vi "Modules Edit.vi"(6 "Queue Ref":T1={"UI"=refnum, "Message"=refnum, "Data"=refnum, "Caller"=refnum, "Name"="000 Common", "Data Path"=path "", "Class Path"=path "", "SubPanel"=refnum, "Project Name"="", "MNT"="", "Title"="", "Data Source"=refnum, "Queue List"={}, "VI"=refnum, "UE"=refnum}, 8 "error in (no error)":errorcluster caption="Error In", 9 "Data":variant, 10 "Operate":string, 11 "ModulesRef":refnum<vi>) -> (0 "error out":errorcluster caption="Error Out")   [LabVIEW 2020]
uses:
  Alin/QMH/000 Module Data Type.ctl
  Alin/QMH/Queue Message.ctl
  0007 Controls/Data Module.ctl
  0007 Controls/Data Modules.ctl
  0007 Controls/Data Element Single.ctl
  Global/Data Global/SDQ Data Type.ctl
  6af73d8b-4b54-4092-88b9-52990f3e3bae.vi
  94913dd2-90ff-4ca1-8781-ffadfa0ced3e.vi
  d649981d-6ad0-461c-86a9-d94ae38d726b.vi
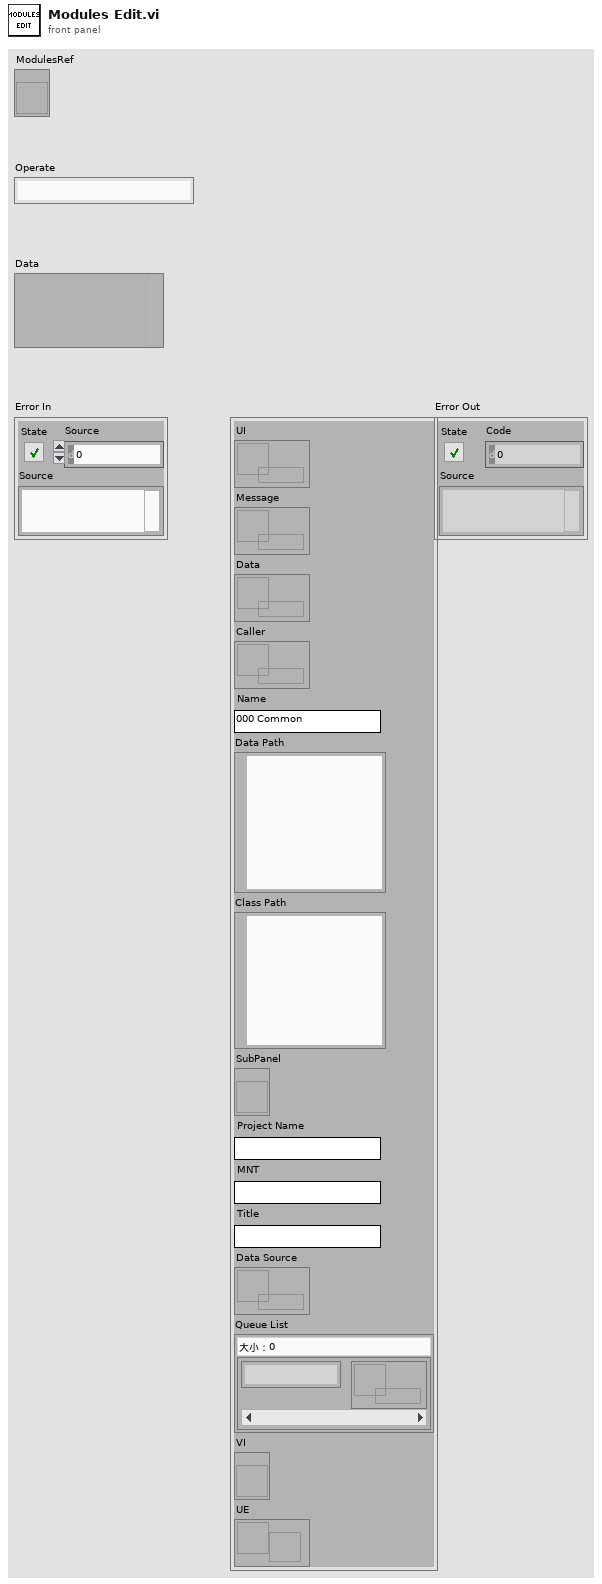
[diagram p1: front panel]
types:
  T1 = typedef "000 Module Data Type.ctl" = cluster{"UI":refnum<queue>, "Message":refnum<queue>, "Data":refnum<queue>, "Caller":refnum<queue>, "Name":string, "Data Path":path, "Class Path":path, "SubPanel":refnum<vi>, "Project Name":string, "MNT":string, "Title":string, "Data Source":refnum<queue>, "Queue List":map{string, refnum<queue>}, "VI":refnum<vi>, "UE":refnum<user-event>}
  T2 = typedef "SDQ Data Type.ctl" = cluster{"CAN Length":string, "CAN Name":string, "CAN ID":string, "CAN Type":string, "Test Item":string, "Byte Order":string, "Instruction":string, "Control Type":string, "Group":string, "Offset":dbl, "Coefficient":dbl, "Write Enable":bool, "Lable Type":string, "Key?":string, "Set Value":string, "Upper":dbl, "Lower":dbl, "Unit":string, "Formula":string, "Test Item Type":string, "Length":i32, "Address":string, "Name":string, "Identifier":string, "Data Type":string, "Enumerate?":string, "Enumerate List":string, "Data":string, "Source":string}
  T3 = cluster{"Receive Data":map{string, T2}, "Queue Ref":T1, "Digit":dbl, "ModulesRef":refnum<vi>, "Index":cluster{"Row":i32, "Colcum":i32, "Digit":dbl}, "Last Index":cluster{"Row":i32, "Colcum":i32, "Digit":dbl}}
  T4 = typedef "Data Module.ctl" = cluster{"Module01":T5, "Module02":T5, "Module03":T5, "Module04":T5, "Module05":T5, "Module06":T5, "Module07":T5, "Module08":T5, "Module09":T5, "Module10":T5, "Module11":T5}
  T5 = typedef "Data Modules.ctl" = cluster{"Names":cluster{"Module Name":string, "Set Value":string, "Real Value":string, "FB Value":string, "Unit":string, "Identifier":string, "IdentifierW":string, "Decimal":string, "AS":bool, "AR":bool, "Con":bool}, "Data":T6[], "Digit":dbl}
  T6 = typedef "Data Element Single.ctl" = cluster{"Name":string, "Set Value":string, "Real Value":string, "FB Value":string, "Unit":string, "Identifier":string, "Write Name":string, "Decimal":u16, "AS":bool, "AR":bool, "ALM":bool, "Up":bool, "Down":bool}
  T7 = cluster{"输出簇":cluster{i32, i32, "Digit":dbl}, "Modules":T4}
  T8 = cluster{"Modules[0]":T5, "Modules[1]":T5, "Modules[2]":T5, "Modules[3]":T5, "Modules[4]":T5, "Modules[5]":T5, "Modules[6]":T5, "Modules[7]":T5, "Modules[8]":T5, "Modules[9]":T5, "Modules[10]":T5}
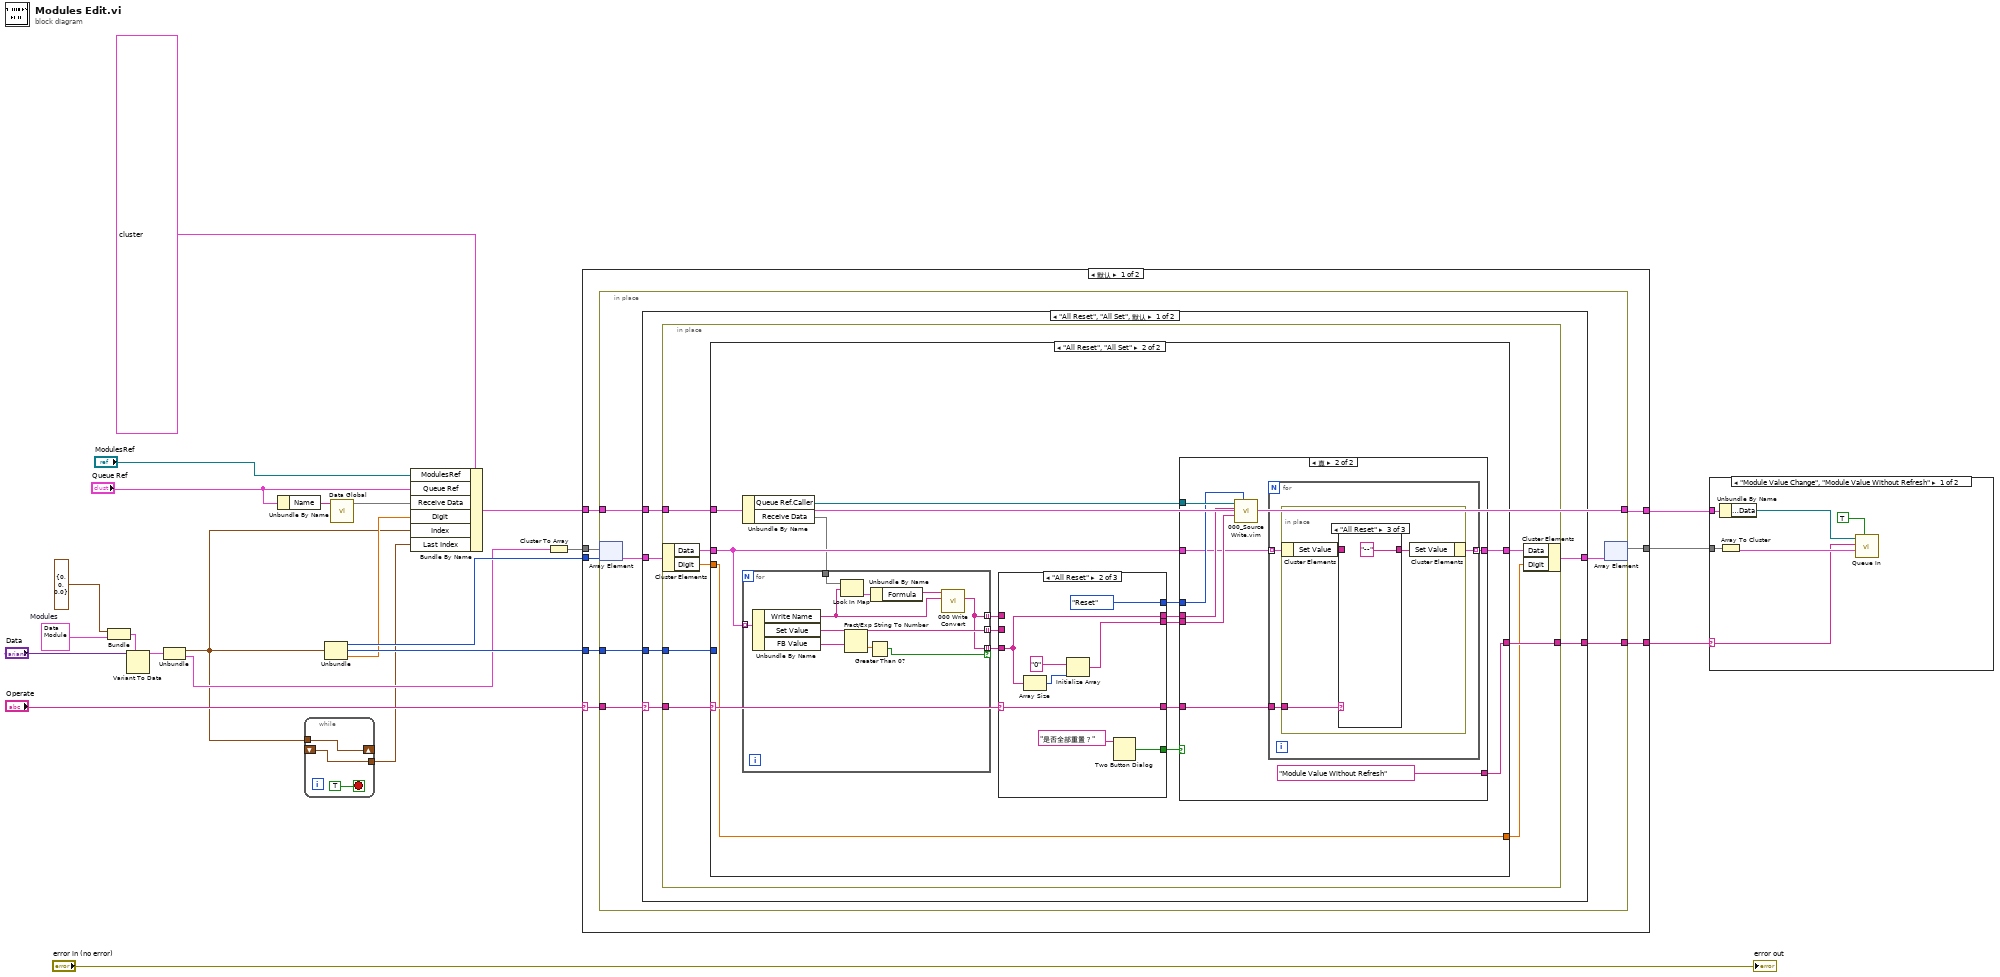
[diagram p0: block diagram]
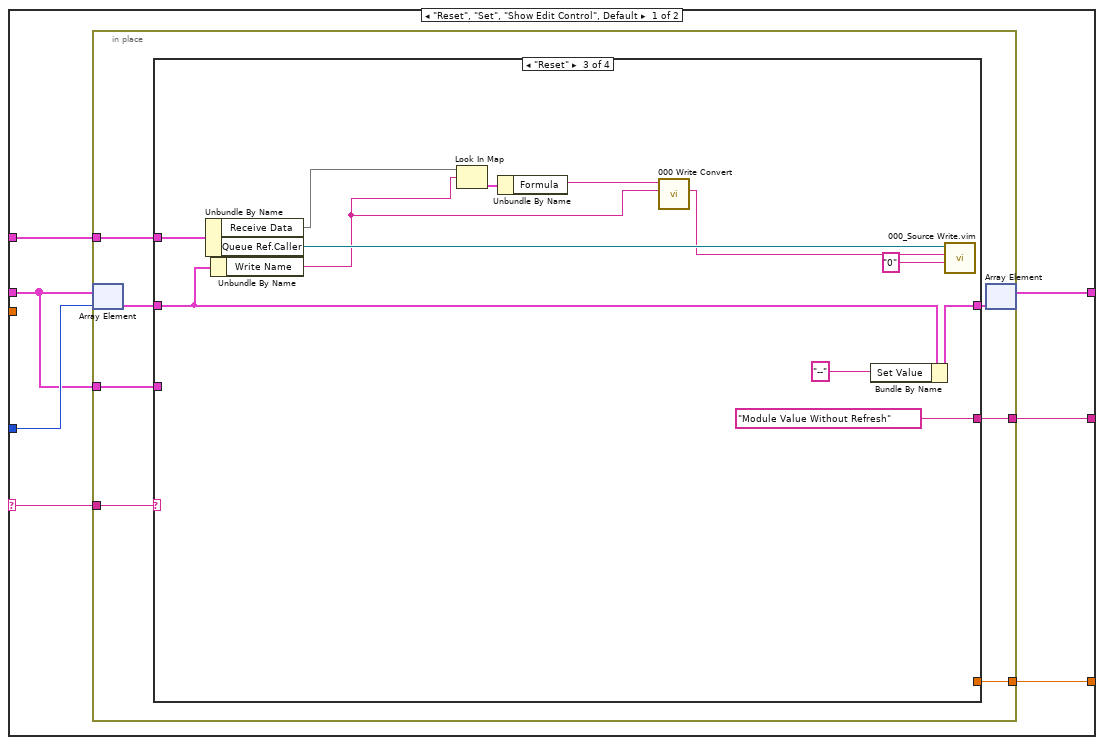
[diagram p2: hidden frame]
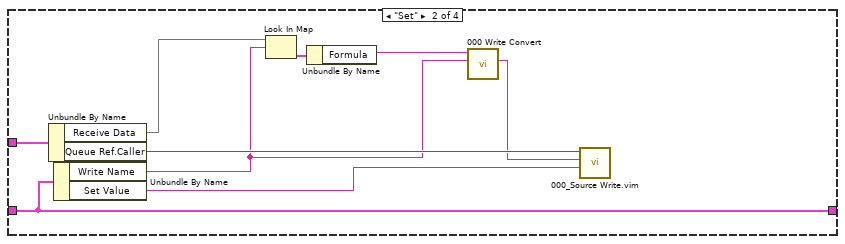
[diagram p4: hidden frame]
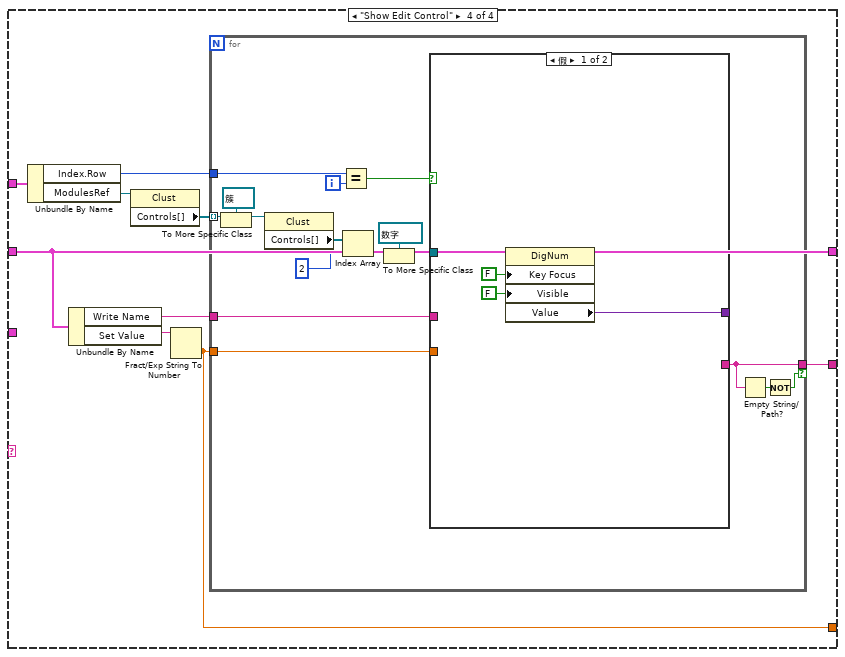
[diagram p5: hidden frame]
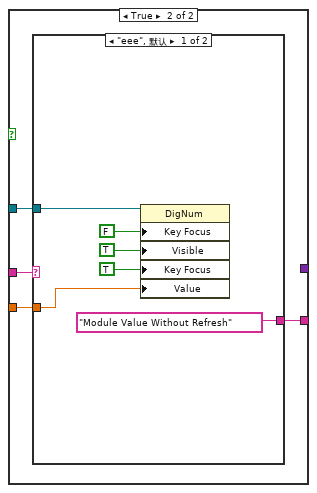
[diagram p6: hidden frame]
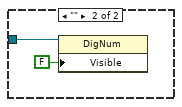
[diagram p7: hidden frame]
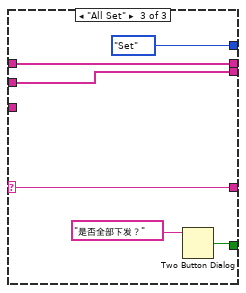
[diagram p12: hidden frame]
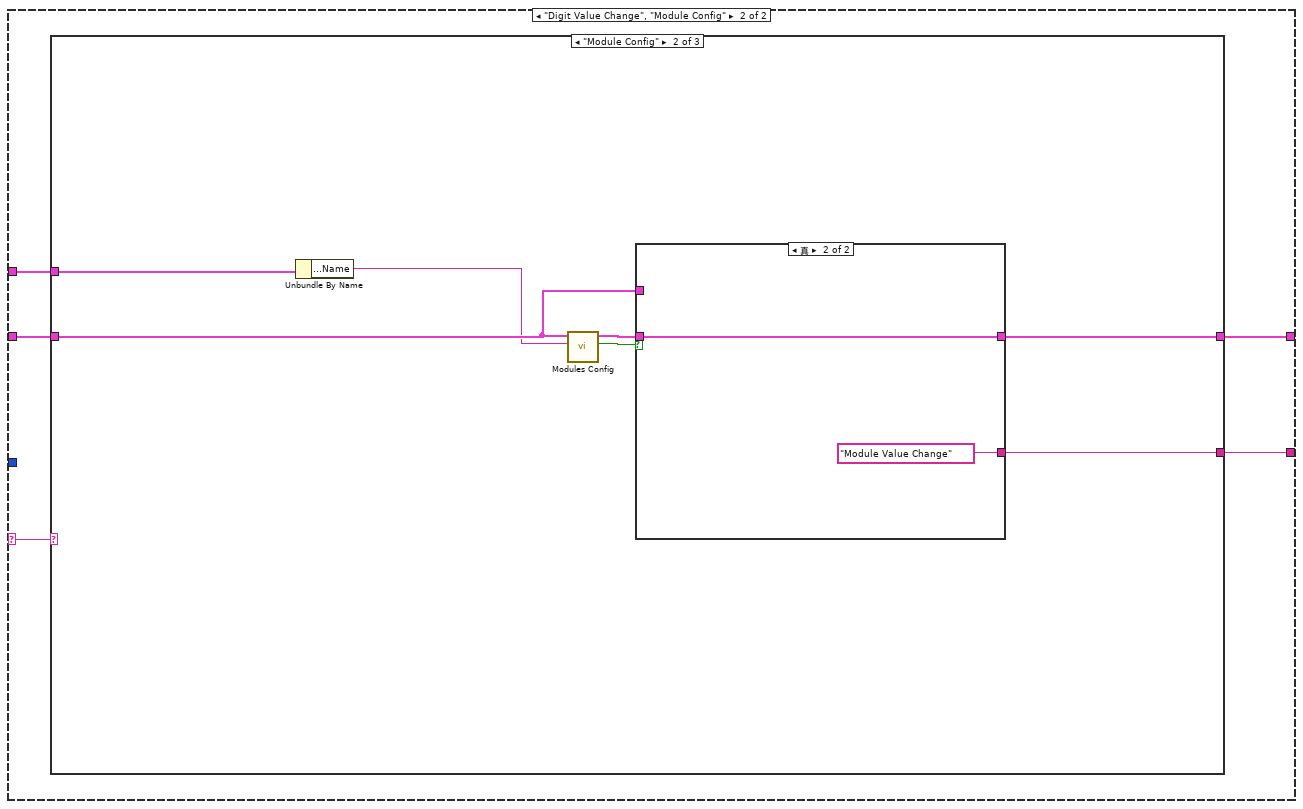
[diagram p13: hidden frame]
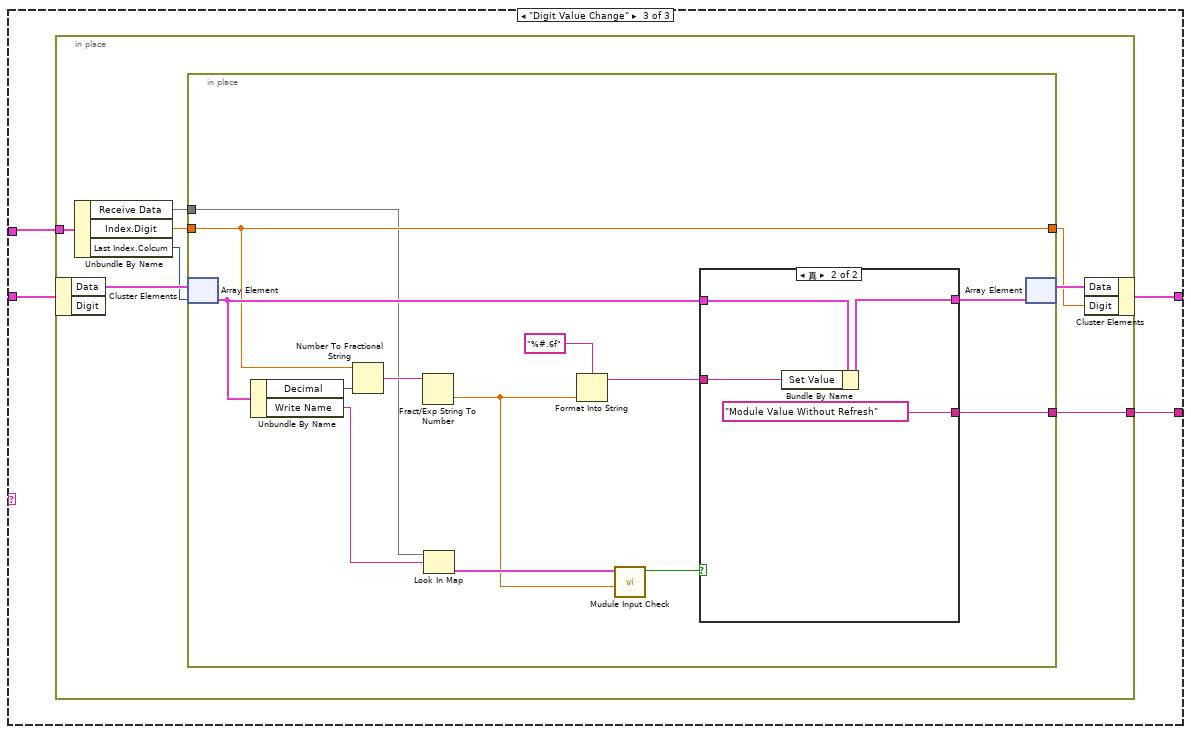
[diagram p16: hidden frame]
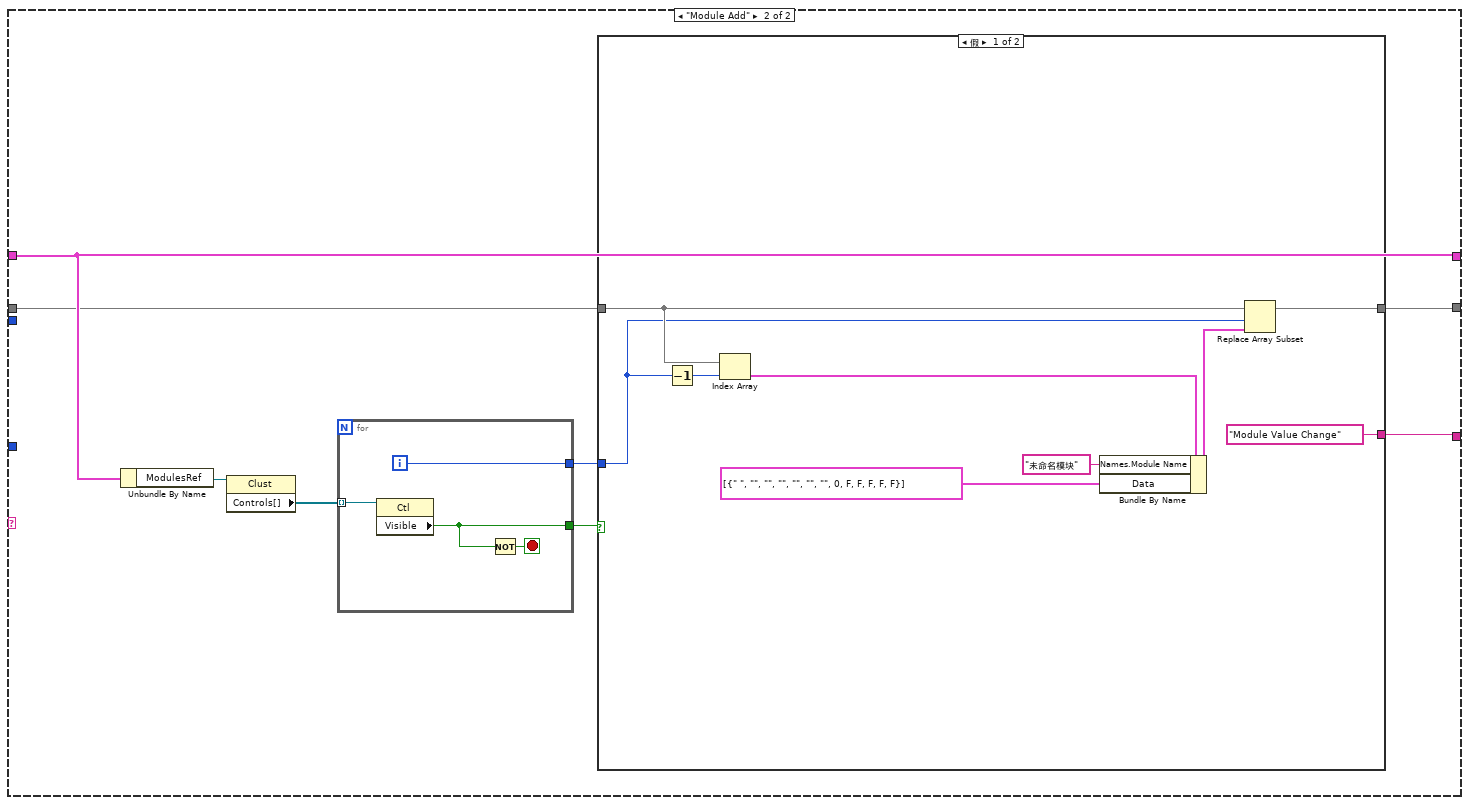
[diagram p18: hidden frame]
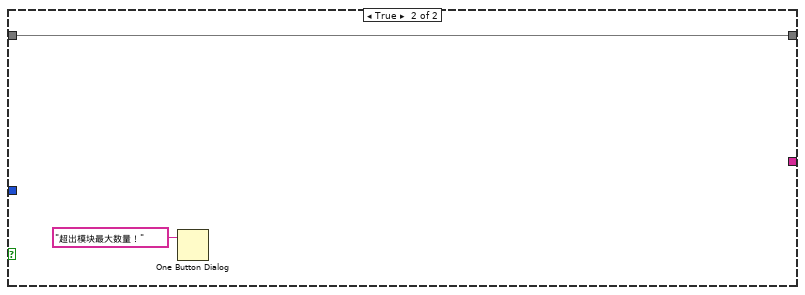
[diagram p19: hidden frame]
diagram:
  w13 = T4 {"Module01"={"Names"={"Module Name"="", "Set Value"="", "Real Value"="", "FB Value"="", "Unit"="", "Identifier"="", "IdentifierW"="写入标识符", "Decimal"="位数", "AS"=FALSE, "AR"=FALSE, "Con"=FALSE}, "Data"=[], "Digit"=0.0}, "Module02"={"Names"={"Module Name"="", "Set Value"="", "Real Value"="", "FB Value"="", "Unit"="", "Identifier"="", "IdentifierW"="写入标识符", "Decimal"="位数", "AS"=FALSE, "AR"=FALSE, "Con"=FALSE}, "Data"=[], "Digit"=0.0}, "Module03"={"Names"={"Module Name"="", "Set Value"="", "Real Value"="", "FB Value"="", "Unit"="", "Identifier"="", "IdentifierW"="写入标识符", "Decimal"="位数", "AS"=FALSE, "AR"=FALSE, "Con"=FALSE}, "Data"=[], "Digit"=0.0}, "Module04"={"Names"={"Module Name"="", "Set Value"="", "Real Value"="", "FB Value"="", "Unit"="", "Identifier"="", "IdentifierW"="写入标识符", "Decimal"="位数", "AS"=FALSE, "AR"=FALSE, "Con"=FALSE}, "Data"=[], "Digit"=0.0}, "Module05"={"Names"={"Module Name"="", "Set Value"="", "Real Value"="", "FB Value"="", "Unit"="", "Identifier"="", "IdentifierW"="写入标识符", "Decimal"="位数", "AS"=FALSE, "AR"=FALSE, "Con"=FALSE}, "Data"=[], "Digit"=0.0}, "Module06"={"Names"={"Module Name"="", "Set Value"="", "Real Value"="", "FB Value"="", "Unit"="", "Identifier"="", "IdentifierW"="写入标识符", "Decimal"="位数", "AS"=FALSE, "AR"=FALSE, "Con"=FALSE}, "Data"=[], "Digit"=0.0}, "Module07"={"Names"={"Module Name"="", "Set Value"="", "Real Value"="", "FB Value"="", "Unit"="", "Identifier"="", "IdentifierW"="写入标识符", "Decimal"="位数", "AS"=FALSE, "AR"=FALSE, "Con"=FALSE}, "Data"=[], "Digit"=0.0}, "Module08"={"Names"={"Module Name"="", "Set Value"="", "Real Value"="", "FB Value"="", "Unit"="", "Identifier"="", "IdentifierW"="写入标识符", "Decimal"="位数", "AS"=FALSE, "AR"=FALSE, "Con"=FALSE}, "Data"=[], "Digit"=0.0}, "Module09"={"Names"={"Module Name"="", "Set Value"="", "Real Value"="", "FB Value"="", "Unit"="", "Identifier"="", "IdentifierW"="写入标识符", "Decimal"="位数", "AS"=FALSE, "AR"=FALSE, "Con"=FALSE}, "Data"=[], "Digit"=0.0}, "Module10"={"Names"={"Module Name"="", "Set Value"="", "Real Value"="", "FB Value"="", "Unit"="", "Identifier"="", "IdentifierW"="写入标识符", "Decimal"="位数", "AS"=FALSE, "AR"=FALSE, "Con"=FALSE}, "Data"=[], "Digit"=0.0}, "Module11"={"Names"={"Module Name"="", "Set Value"="", "Real Value"="", "FB Value"="", "Unit"="", "Identifier"="", "IdentifierW"="写入标识符", "Decimal"="位数", "AS"=FALSE, "AR"=FALSE, "Con"=FALSE}, "Data"=[], "Digit"=0.0}}  # Modules
  n1 = Bundle("输出簇"=cluster{i32, i32, "Digit":dbl} {0, 0, "Digit"=0.0}, "Modules"=w13) -> (w12:T7)  [unwired: 1 in]
  n2 = Variant To Data(type=w12, Variant="Data") -> (data=w14:T7)  [unwired: 1 in, 1 out]
  n3 = Unbundle(w14) -> ("输出簇"=w2:cluster{i32, i32, "Digit":dbl}, "Modules"=w7:T4)
  n4 = Unbundle By Name("Queue Ref") -> ("Name"=w5:string)
  n5 = while {
    shift-right: [w26] -> _
    shift-left: _ -> [w24]
    tunnel: w2 -> [w26]
    tunnel: [w24] -> w1
    stop <- TRUE stop-if-true
  }
  n6 = Unbundle(w2) -> (w16:i32, w19:i32, "Digit"=w3:dbl)
  n7 = call "Data Global.vi"("Name"=w5) -> ("Data Out"=w4:map{string, T2})  [unwired: 7 in, 3 out]
  n8 = Bundle By Name(cluster=T3 {"Receive Data"={}, "Queue Ref"={"UI"=refnum, "Message"=refnum, "Data"=refnum, "Caller"=refnum, "Name"="0001_HZKD_ST01-DSM-002_DataMonitor", "Data Path"=path "D:/NBT/01-Project/02-Processing/NBT-TestPlatform V2/NBT-TestPlatform 20230413_0/Config/NBT/NBT_V1.0.0/Project/0001_HZKD_ST01/04_DataUse/002_DataMonitor.csv", "Class Path"=path "D:/NBT/01-Project/02-Processing/NBT-TestPlatform V2/NBT-TestPlatform 20230413_0/Modules/000 UI/002_Module/002_DataMonitor.vi", "SubPanel"=refnum, "Project Name"="0001_HZKD_ST01", "MNT"="", "Title"="", "Data Source"=refnum, "Queue List"={}, "VI"=refnum, "UE"=refnum}, "Digit"=0.0, "ModulesRef"=refnum, "Index"={"Row"=0, "Colcum"=0, "Digit"=0.0}, "Last Index"={"Row"=0, "Colcum"=0, "Digit"=0.0}}, "ModulesRef"="ModulesRef", "Queue Ref"="Queue Ref", "Receive Data"=w4, "Digit"=w3, "Index"=w2, "Last Index"=w1) -> (w10:T3)
  n9 = Cluster To Array(cluster=w7) -> (array=w23:T5[])
  n10 = case shown="默认" "Operate" {
    selector: "Operate" -> [w31 _]
    tunnel: w23 -> [w34 w239]
    tunnel: [w33 w238] -> w21
    tunnel: w19 -> [w32 _]
    tunnel: w16 -> [w30 _]
    tunnel: w10 -> [w29 w244]
    tunnel: [w28 w244] -> w9
    tunnel: [w27 w237] -> w8
    frame Default {
      n11 = in-place {
        in-place-border: w32 -> [w40]
        in-place-border: w31 -> [w38]
        in-place-border: w29 -> [w37]
        in-place-border: [w37] -> w28
        in-place-border: [w35] -> w27
        n12 = in-place-array #1(w34, w30) -> (w36:T5)
        n13 = case shown="\"All Reset\", \"All Set\", 默认" w38 {
          selector: w38 -> [w44 w192]
          tunnel: w40 -> [w46 _]
          tunnel: [w45 w194] -> w39
          tunnel: w37 -> [w43 w195]
          tunnel: w36 -> [w42 w193]
          tunnel: [w41 w191] -> w35
          frame "All Reset", "All Set", Default {
            n14 = in-place {
              in-place-border: w46 -> [w54]
              in-place-border: w44 -> [w52]
              in-place-border: w43 -> [w49]
              in-place-border: [w48] -> w41
              n15 = in-place-cluster #2(w42) -> ("Data"=w51:T6[], "Digit"=w50:dbl)
              n16 = case shown="\"All Reset\", \"All Set\"" w52 {
                selector: w52 -> [w59 w145]
                tunnel: w54 -> [w61 _]
                tunnel: [w60 w138] -> w53
                tunnel: w51 -> [w58 w139]
                tunnel: w50 -> [_ w135]
                tunnel: w49 -> [w57 w147]
                tunnel: [w56 w136] -> w48
                tunnel: [w55 w135] -> w47
                frame "Reset", "Set", "Show Edit Control", Default {
                  n17 = in-place {
                    in-place-border: w59 -> [w67]
                    in-place-border: w58 -> [w65]
                    in-place-border: w57 -> [w64]
                    in-place-border: [w63] -> w56
                    in-place-border: [w62] -> w55
                    n18 = in-place-array #3(w58, w61) -> (w68:T6)
                    n19 = case shown="\"Reset\"" w67 {
                      tunnel: w68 -> [w69 w76 w85 w95]
                      tunnel: [w69 w76 w90 w95] -> w66
                      tunnel: w65 -> [_ _ _ _]
                      tunnel: w64 -> [_ w78 w86 w99]
                      tunnel: [_ _ "Module Value Without Refresh" w91] -> w63
                      tunnel: [_ _ _ w92] -> w62
                      frame "eee", Default {
                      }
                      frame "Set" {
                        n20 = Unbundle By Name(w78) -> ("Receive Data"=w74:map{string, T2}, "Queue Ref.Caller"=w77:refnum<queue>)
                        n21 = Unbundle By Name(w76) -> ("Write Name"=w71:string, "Set Value"=w75:string)
                        n22 = Look In Map(map=w74, key=w71) -> (value=w73:T2)  [unwired: 1 in, 1 out]
                        n23 = Unbundle By Name(w73) -> ("Formula"=w72:string)
                        n24 = call "000 Write Convert.vi"("Name In"=w71, "Formular"=w72) -> ("Name Out"=w70:string)  [unwired: 9 in]
                        n25 = call "000_Source Write.vim"("Data"=w75, "Name"=w70, "Queue In"=w77) -> ()  [unwired: 6 in, 3 out]
                      }
                      frame "Reset" {
                        n26 = Unbundle By Name(w86) -> ("Receive Data"=w81:map{string, T2}, "Queue Ref.Caller"=w87:refnum<queue>)
                        n27 = Unbundle By Name(w85) -> ("Write Name"=w80:string)
                        n28 = Look In Map(map=w81, key=w80) -> (value=w83:T2)  [unwired: 1 in, 1 out]
                        n29 = Unbundle By Name(w83) -> ("Formula"=w82:string)
                        n30 = call "000 Write Convert.vi"("Name In"=w80, "Formular"=w82) -> ("Name Out"=w79:string)  [unwired: 9 in]
                        n31 = Bundle By Name(cluster=w85, "Set Value"="--") -> (w90:T6)
                        n32 = call "000_Source Write.vim"("Data"="0", "Name"=w79, "Queue In"=w87) -> ()  [unwired: 6 in, 3 out]
                      }
                      frame "Show Edit Control" {
                        n33 = Unbundle By Name(w99) -> ("Index.Row"=w96:i32, "ModulesRef"=w98:refnum<vi>)
                        n34 = Unbundle By Name(w95) -> ("Write Name"=w93:string, "Set Value"=w94:string)
                        n35 = property class="Clust"(reference=w98) -> ("Controls[]"=w97:refnum<vi>[])  [unwired: 1 in, 2 out]
                        n36 = Fract/Exp String To Number(string=w94) -> (number=w92:dbl)  [unwired: 3 in, 1 out]
                        n37 = for {
                          tunnel: w97 -> [w111] mode=indexing
                          tunnel: w96 -> [w109]
                          tunnel: w92 -> [w105]
                          tunnel: w93 -> [w103]
                          tunnel: [w102] -> w91 if=w100
                          i -> [w108]
                          n38 = To More Specific Class(target class=refnum<vi> refnum ("ModulesRef"), reference=w111) -> (specific class reference=w115:refnum<vi>)  [unwired: 1 in, 1 out]
                          n39 = property class="Clust"(reference=w115) -> ("Controls[]"=w114:refnum<vi>[])  [unwired: 1 in, 2 out]
                          n40 = Equal?(x=w109, y=w108) -> (x = y?=w107:bool)
                          n41 = Index Array(array=w114, index=2 ("索引")) -> (element=w110:refnum<vi>)
                          n42 = To More Specific Class(target class=refnum<vi> refnum ("Digit"), reference=w110) -> (specific class reference=w106:refnum<vi>)  [unwired: 1 in, 1 out]
                          n43 = case shown="假" w107 {
                            tunnel: w106 -> [w119 w123]
                            tunnel: w105 -> [_ w122]
                            tunnel: w103 -> [_ w121]
                            tunnel: [_ w120] -> w102
                            tunnel: [w116 _] -> _
                            frame False {
                              n44 = property class="DigNum"(reference=w119, "Key Focus"=FALSE ("键选中"), "Visible"=FALSE ("可见")) -> ("Value"=w116:variant)  [unwired: 1 in, 2 out]
                            }
                            frame True {
                              n45 = case shown="\"eee\", 默认" w121 {
                                tunnel: w123 -> [w127 w130]
                                tunnel: w122 -> [w126 _]
                                tunnel: ["Module Value Without Refresh" _] -> w120
                                frame "eee", Default {
                                n46 = property class="DigNum"(reference=w127, "Key Focus"=FALSE ("键选中"), "Visible"=TRUE ("可见"), "Key Focus"=TRUE ("键选中"), "Value"=w126) -> ()  [unwired: 1 in, 2 out]
                                }
                                frame "" {
                                n47 = property class="DigNum"(reference=w130, "Visible"=FALSE ("可见")) -> ()  [unwired: 1 in, 2 out]
                                }
                              }
                            }
                          }
                          n48 = Empty String/Path?(string/path=w102) -> (empty?=w101:bool)
                          n49 = Not(x=w101) -> (.not. x?=w100:bool)
                        }
                      }
                    }
                    n50 = in-place-array #3(w66) -> (w60:T6[])  [unwired: 1 out]
                  }
                }
                frame "All Reset", "All Set" {
                  n51 = Unbundle By Name(w147) -> ("Queue Ref.Caller"=w146:refnum<queue>, "Receive Data"=w133:map{string, T2})
                  n52 = for {
                    tunnel: w139 -> [w190] mode=indexing
                    tunnel: [w181] -> w144 mode=indexing
                    tunnel: [w183] -> w143 mode=indexing
                    tunnel: [w181] -> w134 mode=indexing if=w188
                    tunnel: w133 -> [w184]
                    n53 = Unbundle By Name(w190) -> ("Write Name"=w182:string, "Set Value"=w183:string, "FB Value"=w187:string)
                    n54 = Look In Map(map=w184, key=w182) -> (value=w186:T2)  [unwired: 1 in, 1 out]
                    n55 = Fract/Exp String To Number(string=w187) -> (number=w189:dbl)  [unwired: 3 in, 1 out]
                    n56 = Greater Than 0?(x=w189) -> (x > 0?=w188:bool)
                    n57 = Unbundle By Name(w186) -> ("Formula"=w185:string)
                    n58 = call "000 Write Convert.vi"("Name In"=w182, "Formular"=w185) -> ("Name Out"=w181:string)  [unwired: 9 in]
                  }
                  n59 = case shown="\"All Reset\"" w145 {
                    selector: w145 -> [w166 w170 w177]
                    tunnel: w144 -> [_ _ w180]
                    tunnel: w143 -> [_ _ w179]
                    tunnel: [_ w169 w180] -> w142
                    tunnel: [_ w172 w179] -> w141
                    tunnel: [_ enum16{"Set", "Reset"}."Reset" ("Operate") enum16{"Set", "Reset"}."Set" ("Operate")] -> w140
                    tunnel: [w166 w170 w177] -> w137
                    tunnel: w134 -> [_ w169 _]
                    tunnel: [_ w167 w176] -> w132
                    frame "eee", Default {
                    }
                    frame "All Reset" {
                      n60 = Array Size(array=w169) -> (size(s)=w173:i32)
                      n61 = Initialize Array("0", w173) -> (w172:string[])
                      n62 = Two Button Dialog(message="是否全部重置？") -> (T button?=w167:bool)  [unwired: 2 in]
                    }
                    frame "All Set" {
                      n63 = Two Button Dialog(message="是否全部下发？") -> (T button?=w176:bool)  [unwired: 2 in]
                    }
                  }
                  n64 = case shown="真" w132 {
                    tunnel: w146 -> [_ w156]
                    tunnel: w142 -> [_ w155]
                    tunnel: w141 -> [_ w154]
                    tunnel: w140 -> [_ w153]
                    tunnel: w139 -> [w148 w152]
                    tunnel: [w148 w151] -> w138
                    tunnel: w137 -> [_ w150]
                    tunnel: [_ "Module Value Without Refresh"] -> w136
                    frame False {
                    }
                    frame True {
                      n65 = call "000_Source Write.vim"("Operate"=w153, "Data"=w154, "Name"=w155, "Queue In"=w156) -> ()  [unwired: 5 in, 3 out]
                      n66 = for {
                        tunnel: w152 -> [w159] mode=indexing
                        tunnel: [w158] -> w151 mode=indexing
                        tunnel: w150 -> [w157]
                        n67 = in-place {
                          in-place-border: w157 -> [w162]
                          n68 = in-place-cluster #4(w159) -> ("Set Value"=w161:string)
                          n69 = case shown="\"All Reset\"" w162 {
                            tunnel: w161 -> [w163 w164 _]
                            tunnel: [w163 w164 "--" ("Name")] -> w160
                            frame "eee", Default {
                            }
                            frame "All Set" {
                            }
                            frame "All Reset" {
                            }
                          }
                          n70 = in-place-cluster #4("Set Value"=w160) -> (w158:T6)
                        }
                      }
                    }
                  }
                }
              }
              n71 = in-place-cluster #2("Data"=w53, "Digit"=w47) -> (w45:T5)
            }
          }
          frame "Digit Value Change", "Module Config" {
            n72 = case shown="\"Module Config\"" w192 {
              tunnel: w195 -> [_ w203 w208]
              tunnel: [w196 w200 w209] -> w194
              tunnel: w193 -> [w196 w199 w210]
              tunnel: [_ w198 w207] -> w191
              frame "eee", Default {
              }
              frame "Module Config" {
                n73 = Unbundle By Name(w203) -> ("Queue Ref.Name"=w197:string)
                n74 = call "Modules Config.vi"("Name"=w197, "Module In"=w199) -> ("OK？"=w202:bool, "Module Out"=w201:T5)  [unwired: 8 in]
                n75 = case shown="真" w202 {
                  tunnel: w201 -> [_ w206]
                  tunnel: [w204 w206] -> w200
                  tunnel: w199 -> [w204 _]
                  tunnel: [_ "Module Value Change"] -> w198
                  frame False {
                  }
                  frame True {
                  }
                }
              }
              frame "Digit Value Change" {
                n76 = in-place {
                  in-place-border: w208 -> [w217]
                  in-place-border: [w213] -> w207
                  n77 = in-place-cluster #5(w210) -> ("Data"=w218:T6[])  [unwired: 1 out]
                  n78 = Unbundle By Name(w217) -> ("Receive Data"=w211:map{string, T2}, "Index.Digit"=w215:dbl, "Last Index.Colcum"=w216:i32)
                  n79 = in-place {
                    in-place-border: w215 -> [w227]
                    in-place-border: [w229] -> w213
                    in-place-border: [w227] -> w212
                    in-place-border: w211 -> [w223]
                    n80 = in-place-array #6(w218, w216) -> (w231:T6)
                    n81 = Unbundle By Name(w231) -> ("Decimal"=w226:u16, "Write Name"=w222:string)
                    n82 = Number To Fractional String(number=w227, precision (6)=w226) -> (F-format string=w225:string)  [unwired: 2 in]
                    n83 = Fract/Exp String To Number(string=w225) -> (number=w220:dbl)  [unwired: 3 in, 1 out]
                    n84 = Look In Map(map=w223, key=w222) -> (value=w221:T2)  [unwired: 1 in, 1 out]
                    n85 = Format Into String(format string="%#.6f" ("格式字符串"), w220) -> (resulting string=w224:string)  [unwired: 2 in, 1 out]
                    n86 = call "Mudule Input Check.vi"("Data In"=w220, "Value"=w221) -> ("OK?"=w219:bool)  [unwired: 9 in]
                    n87 = case shown="真" w219 {
                      tunnel: w231 -> [w232 w236]
                      tunnel: [w232 w235] -> w230
                      tunnel: [_ "Module Value Without Refresh"] -> w229
                      tunnel: w224 -> [_ w233]
                      frame False {
                      }
                      frame True {
                        n88 = Bundle By Name(cluster=w236, "Set Value"=w233) -> (w235:T6)
                      }
                    }
                    n89 = in-place-array #6(w230) -> (w214:T6[])  [unwired: 1 out]
                  }
                  n90 = in-place-cluster #5("Data"=w214, "Digit"=w212) -> (w209:T5)
                }
              }
            }
          }
        }
        n91 = in-place-array #1(w39) -> (w33:T5[])  [unwired: 1 out]
      }
    }
    frame "Module Add" {
      n92 = Unbundle By Name(w244) -> ("ModulesRef"=w243:refnum<vi>)
      n93 = property class="Clust"(reference=w243) -> ("Controls[]"=w242:refnum<vi>[])  [unwired: 1 in, 2 out]
      n94 = for {
        tunnel: w242 -> [w259] mode=indexing
        tunnel: [w257] -> w241
        tunnel: [w256] -> w240
        i -> [w256]
        stop <- w258 stop-if-true
        n95 = property class="Ctl"(reference=w259) -> ("Visible"=w257:bool)  [unwired: 1 in, 2 out]
        n96 = Not(x=w257) -> (.not. x?=w258:bool)
      }
      n97 = case shown="假" w241 {
        tunnel: w240 -> [w250 _]
        tunnel: w239 -> [w253 w254]
        tunnel: [w252 w254] -> w238
        tunnel: ["Module Value Change" _] -> w237
        frame False {
          n98 = Decrement(x=w250) -> (x-1=w245:i32)
          n99 = Index Array(array=w253, index=w245) -> (element=w251:T5)
          n100 = Bundle By Name(cluster=w251, "Names.Module Name"="未命名模块", "Data"=T6[] [{"Name"=" ", "Set Value"="", "Real Value"="", "FB Value"="", "Unit"="", "Identifier"="", "Write Name"="", "Decimal"=0, "AS"=FALSE, "AR"=FALSE, "ALM"=FALSE, "Up"=FALSE, "Down"=FALSE}]) -> (w249:T5)
          n101 = Replace Array Subset(array=w253, new element=w249, index=w250) -> (w252:T5[])
        }
        frame True {
          n102 = One Button Dialog(message="超出模块最大数量！" ("消息")) -> ()  [unwired: 1 in, 1 out]
        }
      }
    }
  }
  n103 = case shown="\"Module Value Change\", \"Module Value Without Refresh\"" w8 {
    selector: w8 -> [w261 _]
    tunnel: w21 -> [w265 _]
    tunnel: w9 -> [w263 _]
    frame "Module Value Change", "Module Value Without Refresh" {
      n104 = Unbundle By Name(w263) -> ("Queue Ref.Data"=w262:refnum<queue>)
      n105 = Array To Cluster(array=w265) -> (cluster=w264:T8)
      n106 = call "Queue In.vi"("First"=TRUE, "Data"=w264, "Message"=w261, "Queue In"=w262) -> ()  [unwired: 6 in, 2 out]
    }
    frame "", Default {
    }
  }
  "error out" <- "error in (no error)"
